vi "SetClassCtrl.vi"(8 "error in (no error)":errorcluster caption="entrée d'erreur (pas d'erreur)", 10 "ClassCtrlRef":refnum<vi>, 11 "DefaultDev en entrée":refnum<class "SR530.lvclass"> caption="DNL_LabVIEW Object in") -> (0 "error out":errorcluster caption="sortie d'erreur", 3 "DefaultDev en sortie":refnum<class "SR530.lvclass"> caption="DNL_LabVIEW Object out")   [LabVIEW 2019, in "SR530.lvclass"]
uses:
  SR530.lvclass
  BaseDevice/BaseDevice.lvclass
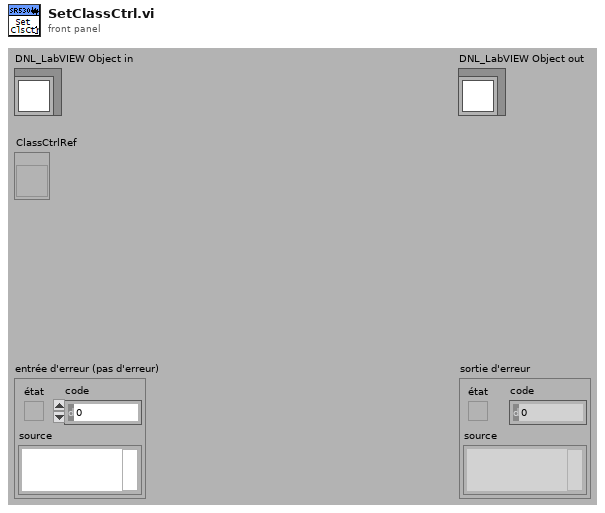
[diagram p1: front panel]
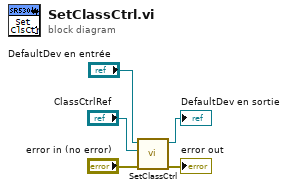
[diagram p0: block diagram]
diagram:
  n1 = call-parent "SetClassCtrl.vi"("error in (no error)"="error in (no error)", "ClassCtrlRef"="ClassCtrlRef", "BaseDevice en entrée"="DefaultDev en entrée") -> ("error out"=→"error out":errorcluster, "BaseDevice en sortie"=→"DefaultDev en sortie":refnum<class "SR530.lvclass">)  [unwired: 7 in]
